vi "Calibration Analysis.vi"(8 "error in (no error)":errorcluster, 11 "Message Queues":T1) -> (0 "error IO":errorcluster, 3 "Results":string[][](array[string]))   [LabVIEW 2026, in "Database.lvlib"]
uses:
  Database.lvlib
  support/Architecture/Message Queue/Message Cluster.ctl
  support/Architecture/Message Queue/Message Queue.lvlib
  support/Architecture/Message Queue/All Message Queues.ctl
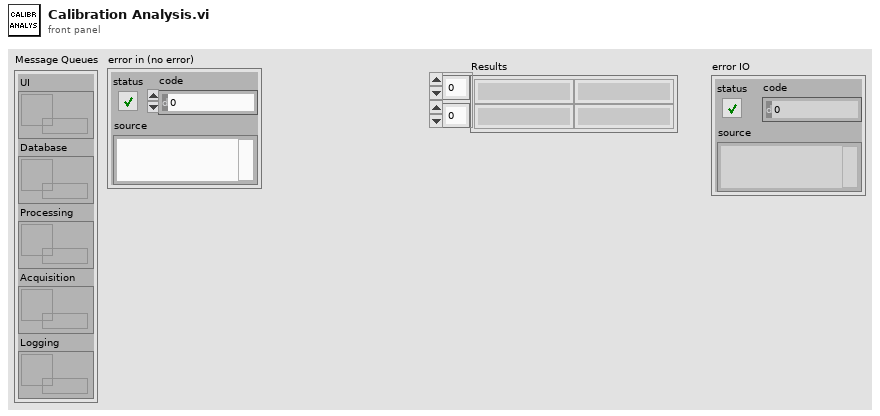
[diagram p1: front panel]
types:
  T1 = typedef "Message Queue.lvlib/All Message Queues.ctl" = cluster{"UI":refnum<queue>, "Database":refnum<queue>, "Processing":refnum<queue>, "Acquisition":refnum<queue>, "Logging":refnum<queue>}
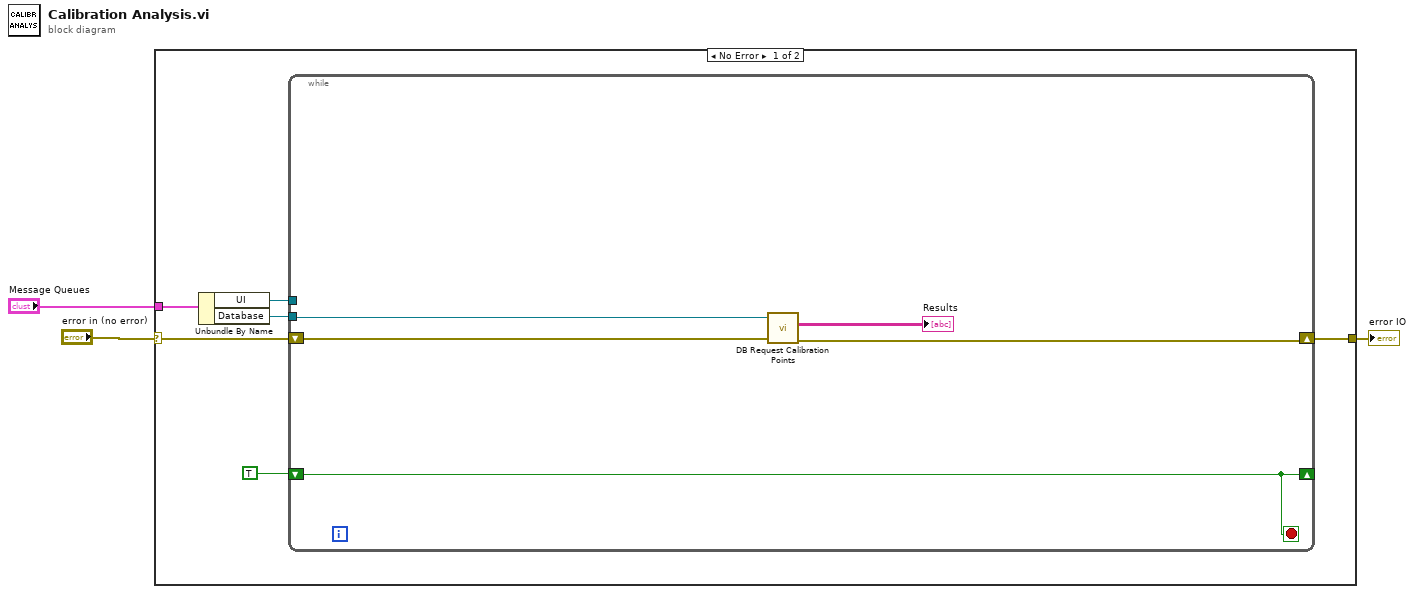
[diagram p0: block diagram]
diagram:
  n1 = case shown="No Error" "error in (no error)" {
    selector: "error in (no error)" -> [w7 w15]
    tunnel: "Message Queues" -> [w9 _]
    tunnel: [w4 w15] -> w1
    frame No Error {
      n2 = Unbundle By Name(w9) -> ("UI"=w6:refnum<queue>, "Database"=w8:refnum<queue>)
      n3 = while {
        tunnel: w8 -> [w13]
        tunnel: w6 -> [_]
        shift-right: [w10] -> w4
        shift-left: w7 -> [w11]
        shift-right: [w14] -> _
        shift-left: TRUE -> [w14]
        stop <- w14 stop-if-true
        n4 = call "DB Request Calibration Points.vi"("error in (no error)"=w11, "Database in"=w13) -> ("error out"=w10:errorcluster, "Results"=→"Results":string[][])  [unwired: 7 in, 1 out]
      }
    }
    frame Error {
    }
  }
  "error IO" <- w1
